vi "Get File.vi"(8 "error in (no error)":errorcluster, 11 "Action?":enum16{"Initialize", "Get Path"}(ring)=enum."Get Path") -> (0 "error out":errorcluster, 3 "File Paths":T1)   [LabVIEW 2021]
uses:
  C:/Users/enProducts/Downloads/KIA_Enproducts/KIA_Enproducts/File Management/File Paths.ctl
  C:/Users/enProducts/Downloads/KIA_Enproducts/KIA_Enproducts/Configuration/Controls/Station Type.ctl
  C:/Users/enProducts/Downloads/KIA_Enproducts/KIA_Enproducts/Configuration/Controls/Part Model.ctl
  75e90ee6-2d5c-4f5d-b705-7a343c88252b.vi
  21bdf65a-1fe2-460d-81cb-cb516824f2e6.vi
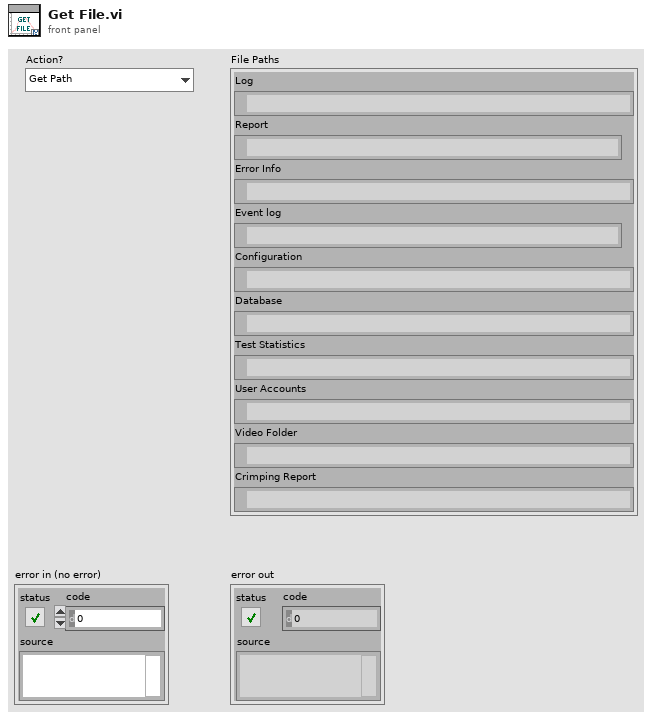
[diagram p1: front panel]
types:
  T1 = typedef "File Paths.ctl" = cluster{"Log":path, "Report":path, "Error Info":path, "Event log":path, "Configuration":path, "Database":path, "Test Statistics":path, "User Accounts":path, "Video Folder":path, "Crimping Report":path}
  T2 = typedef "Part Model.ctl" = enum16{"KIA"}
  T3 = typedef "Station Type.ctl" = enum16{"None", "Station01", "Station02", "Station03", "Station04", "Station05", "Station06", "Station07", "Station08", "Station09", "Station10", "Station11", "Station12", "Station13", "Station14", "Station15", "Station16", "Station17", "Station18", "Station19"}
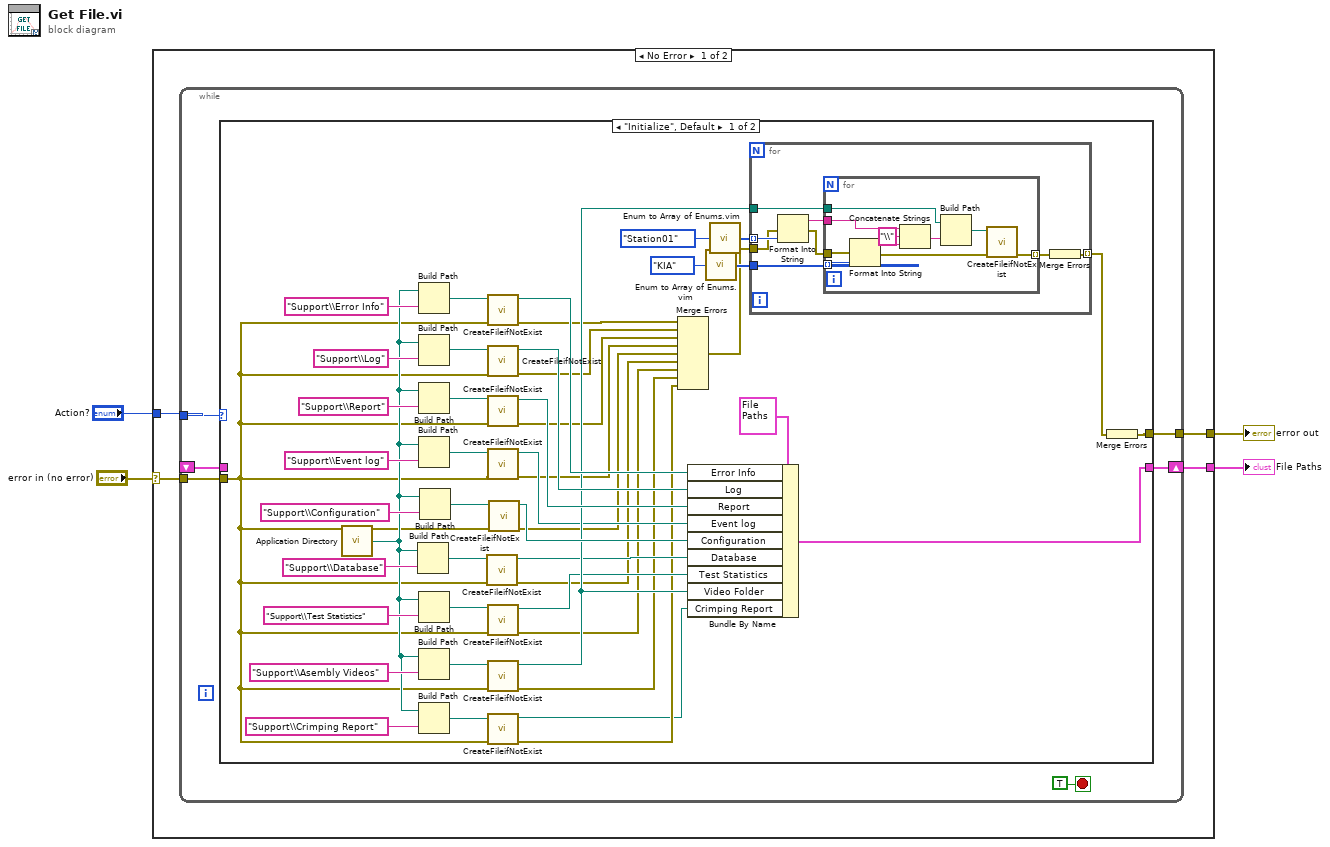
[diagram p0: block diagram]
diagram:
  n1 = case shown="No Error" "error in (no error)" {
    selector: "error in (no error)" -> [w7 w82]
    tunnel: [w6 w82] -> w4
    tunnel: "Action?" -> [w8 _]
    tunnel: [w5 _] -> w1
    frame No Error {
      n2 = while {
        shift-right: [w12] -> w5
        shift-left: _ -> [w11]
        tunnel: w8 -> [w13]
        tunnel: w7 -> [w10]
        tunnel: [w9] -> w6
        stop <- TRUE stop-if-true
        n3 = case shown="\"Initialize\", Default" w13 {
          tunnel: [w60 w81] -> w12
          tunnel: w11 -> [_ w81]
          tunnel: w10 -> [w30 w80]
          tunnel: [w17 w80] -> w9
          frame "Initialize", Default {
            n4 = call <vilib>:"Application Directory.vi"() -> ("Application Directory"=w46:path)
            n5 = Build Path(base path=w46, name or relative path="Support\\Database") -> (appended path=w34:path)
            n6 = Build Path(base path=w46, name or relative path="Support\\Error Info") -> (appended path=w44:path)
            n7 = Build Path(base path=w46, name or relative path="Support\\Log") -> (appended path=w43:path)
            n8 = Build Path(base path=w46, name or relative path="Support\\Report") -> (appended path=w41:path)
            n9 = Build Path(base path=w46, name or relative path="Support\\Event log") -> (appended path=w32:path)
            n10 = Build Path(base path=w46, name or relative path="Support\\Test Statistics") -> (appended path=w35:path)
            n11 = Build Path(base path=w46, name or relative path="Support\\Asembly Videos") -> (appended path=w39:path)
            n12 = Build Path(base path=w46, name or relative path="Support\\Crimping Report") -> (appended path=w37:path)
            n13 = Build Path(base path=w46, name or relative path="Support\\Configuration") -> (appended path=w55:path)
            n14 = call "CreateFileifNotExist.vi"("error in (no error)"=w30, "file path in"=w34) -> ("error out"=w22:errorcluster, "File path out"=w33:path)  [unwired: 8 in]
            n15 = call "CreateFileifNotExist.vi"("error in (no error)"=w30, "file path in"=w44) -> ("error out"=w27:errorcluster, "File path out"=w45:path)  [unwired: 8 in]
            n16 = call "CreateFileifNotExist.vi"("error in (no error)"=w30, "file path in"=w43) -> ("error out"=w26:errorcluster, "File path out"=w42:path)  [unwired: 8 in]
            n17 = call "CreateFileifNotExist.vi"("error in (no error)"=w30, "file path in"=w41) -> ("error out"=w25:errorcluster, "File path out"=w40:path)  [unwired: 8 in]
            n18 = call "CreateFileifNotExist.vi"("error in (no error)"=w30, "file path in"=w32) -> ("error out"=w24:errorcluster, "File path out"=w31:path)  [unwired: 8 in]
            n19 = call "CreateFileifNotExist.vi"("error in (no error)"=w30, "file path in"=w35) -> ("error out"=w21:errorcluster, "File path out"=w36:path)  [unwired: 8 in]
            n20 = call "CreateFileifNotExist.vi"("error in (no error)"=w30, "file path in"=w39) -> ("error out"=w20:errorcluster, "File path out"=w38:path)  [unwired: 8 in]
            n21 = call "CreateFileifNotExist.vi"("error in (no error)"=w30, "file path in"=w37) -> ("error out"=w19:errorcluster, "File path out"=w15:path)  [unwired: 8 in]
            n22 = call "CreateFileifNotExist.vi"("error in (no error)"=w30, "file path in"=w55) -> ("error out"=w23:errorcluster, "File path out"=w52:path)  [unwired: 8 in]
            n23 = Merge Errors(w27, w26, w25, w24, w23, w22, w21, w20, w19) -> (w18:errorcluster)
            n24 = Bundle By Name(cluster=T1 {"Log"=path "", "Report"=path "", "Error Info"=path "", "Event log"=path "", "Configuration"=path "", "Database"=path "", "Test Statistics"=path "", "User Accounts"=path "", "Video Folder"=path "", "Crimping Report"=path ""} ("File Paths"), "Error Info"=w45, "Log"=w42, "Report"=w40, "Event log"=w31, "Configuration"=w52, "Database"=w33, "Test Statistics"=w36, "Video Folder"=w38, "Crimping Report"=w15) -> (w60:T1)
            n25 = call "Enum to Array of Enums.vim"("enum"=Part_Model."KIA" ("Model")) -> ("array of enums"=w29:T2[])
            n26 = call "Enum to Array of Enums.vim"("enum"=Station_Type."Station01" ("Station Info")) -> ("array of enums"=w49:T3[])
            n27 = for {
              tunnel: w49 -> [w65] mode=indexing
              tunnel: w38 -> [w69]
              tunnel: w29 -> [w68]
              tunnel: w18 -> [w64]
              tunnel: [w66] -> w16 mode=indexing
              n28 = Format Into String(error in=w64, w65) -> (resulting string=w62:string, error out=w63:errorcluster)  [unwired: 2 in]
              n29 = for {
                tunnel: w68 -> [w74] mode=indexing
                tunnel: w69 -> [w79]
                tunnel: [w76] -> w67 mode=indexing
                tunnel: w63 -> [w73]
                tunnel: w62 -> [w71]
                n30 = Format Into String(error in=w73, w74) -> (resulting string=w75:string, error out=w77:errorcluster)  [unwired: 2 in]
                n31 = Concatenate Strings(w71, "\\" ("string"), w75) -> (w72:string)
                n32 = Build Path(base path=w79, name or relative path=w72) -> (appended path=w78:path)
                n33 = call "CreateFileifNotExist.vi"("error in (no error)"=w77, "file path in"=w78) -> ("error out"=w76:errorcluster)  [unwired: 8 in, 1 out]
              }
              n34 = Merge Errors(w67) -> (w66:errorcluster)
            }
            n35 = Merge Errors(w16) -> (w17:errorcluster)
          }
          frame "Get Path" {
          }
        }
      }
    }
    frame Error {
    }
  }
  "error out" <- w4
  "File Paths" <- w1
